vi "_Raise StatusBarTextChanged.vi"(4 "WebView2.lvlib:WebView2 Control.lvclass":refnum<class "WebView2 Control.lvclass">, 5 "Event Data":cluster{"sender":refnum<k24>, "e":refnum<k24>}, 6 "Control Ref":refnum<k24>, 7 "Event Common Data":T1) -> ()   [LabVIEW 2025, in "WebView2.lvlib" / "WebView2 Control.lvclass"]
uses:
  WebView2 Control.lvclass
  E:/Labview/LV 2023/PPL/PPL Builder/Libs/LV-WebView2/Source/Libs/Microsoft.Web.WebView2.Core.dll
  Libs/Microsoft.Web.WebView2.Core.dll
  WebView2 Control.lvclass/WebView2 Control.ctl
  WebView2 Event Filter Interface/WebView2 Event Filter Interface.lvclass
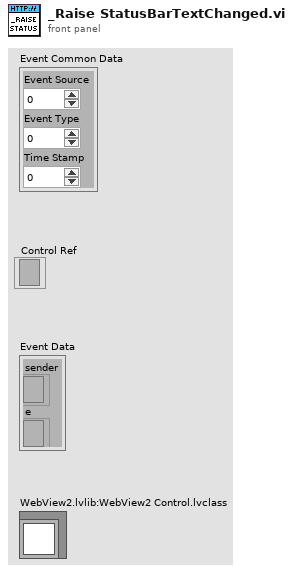
[diagram p1: front panel]
types:
  T1 = cluster{"Event Source":i32, "Event Type":u32, "Time Stamp":u32}
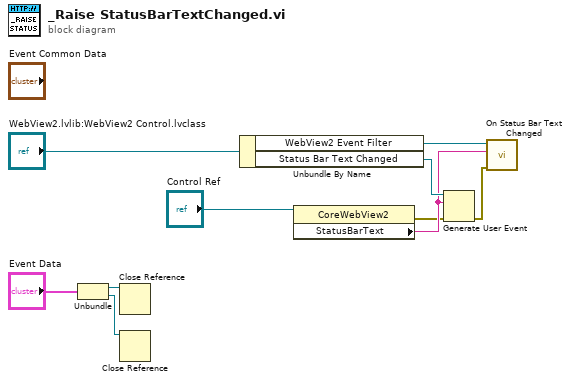
[diagram p0: block diagram]
diagram:
  n1 = Unbundle("Event Data") -> ("sender"=w6:refnum<k24>, "e"=w5:refnum<k24>)
  n2 = Close Reference(reference=w6) -> ()  [unwired: 1 in, 1 out]
  n3 = Close Reference(reference=w5) -> ()  [unwired: 1 in, 1 out]
  n4 = Unbundle By Name("WebView2.lvlib:WebView2 Control.lvclass") -> ("WebView2 Event Filter"=w4:refnum<class "WebView2 Event Filter Interface.lvclass">, "Status Bar Text Changed"=w8:refnum<user-event>)
  n5 = property class="CoreWebView2"(reference="Control Ref") -> (error out=w2:errorcluster, "StatusBarText"=w3:string)  [unwired: 1 in, 1 out]
  n6 = Generate User Event(user event=w8, event data cluster=w3, error in=w2) -> (error out=w1:errorcluster)  [unwired: 1 in, 1 out]
  n7 = call-dynamic "On Status Bar Text Changed.vi"("error in (no error)"=w1, "Text"=w3, "WebView2 Event Filter Interface in"=w4) -> ()  [unwired: 7 in, 2 out]
